vi "Get Data and Log.vi"() -> ()   [LabVIEW 2016]
uses:
  <vilib>/Utility/sysdir.llb/System Directory Type.ctl
  <vilib>/Rock Robotics/Network Tables/NT Read Numeric Array.vi
  <vilib>/Utility/file.llb/Write Delimited Spreadsheet (DBL).vi
panel:
  in  "Mode":T1(ring)=enum."Auto Disabled"
  out "appended path":path
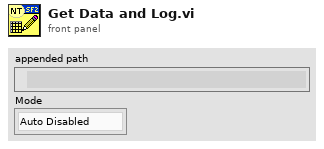
[diagram p1: front panel]
types:
  T1 = enum8{"Tele-Op Disabled", "Tele-Op Enabled", "Auto Disabled", "Auto Enabled", "Test Disabled", "Test Enabled", "Disconnected", "No Code", "E-Stop"}
  T2 = enum16{"open", "replace", "create", "open or create", "replace or create", "replace or create with confirmation"}
  T3 = typedef "System Directory Type.ctl" = i32
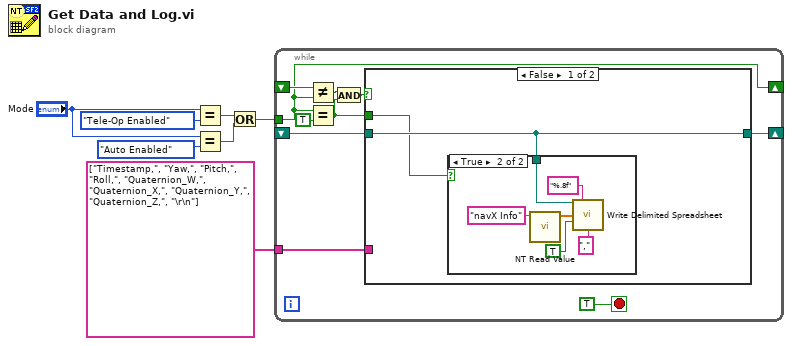
[diagram p0: block diagram]
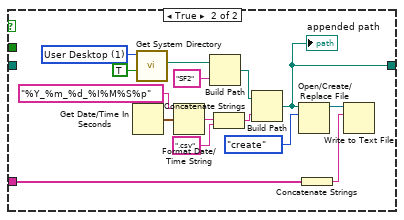
[diagram p3: hidden frame]
diagram:
  n1 = Equal?(x="Mode", y=T1."Tele-Op Enabled") -> (x = y?=w4:bool)
  n2 = Equal?(x="Mode", y=T1."Auto Enabled") -> (x = y?=w3:bool)
  n3 = Or(x=w4, y=w3) -> (x .or. y?=w2:bool)
  n4 = while {
    shift-right: [w15] -> _
    shift-left: _ -> [w16]
    tunnel: w2 -> [w12]
    shift-right: [w12] -> _
    shift-left: _ -> [w14]
    tunnel: string[] ["Timestamp,", "Yaw,", "Pitch,", "Roll,", "Quaternion_W,", "Quaternion_X,", "Quaternion_Y,", "Quaternion_Z,", "\r\n"] -> [w8]
    stop <- TRUE stop-if-true
    n5 = Not Equal?(x=w14, y=w12) -> (x != y?=w13:bool)
    n6 = Equal?(x=w12, y=TRUE) -> (x = y?=w9:bool)
    n7 = And(x=w13, y=w9) -> (x .and. y?=w10:bool)
    n8 = case shown="False" w10 {
      tunnel: [w19 w26] -> w15
      tunnel: w16 -> [w19 _]
      tunnel: w9 -> [w18 _]
      tunnel: w8 -> [_ w31]
      frame False {
        n9 = case shown="True" w18 {
          tunnel: w19 -> [_ w22]
          frame False {
          }
          frame True {
            n10 = call-poly <vilib>:"NT Read Value.vi"("Name"="navX Info") -> ("Numeric Array"=w21:dbl[])  [unwired: 9 in, 1 out]
            n11 = call-poly <vilib>:"Write Delimited Spreadsheet.vi"("file path (dialog if empty)"=w22, "format (%.3f)"="%.8f", "1D data"=w21, "append to file? (new file:F)"=TRUE, "delimiter (\\t)"="," ("delimiter (\\t)")) -> ()  [unwired: 9 in, 2 out]
          }
        }
      }
      frame True {
        w36 = T3 1 items=["User Home"=0, "User Desktop"=1, "User Documents"=2, "User Application Data"=3, "User Preferences"=4, "User Temporary"=5, "Public Documents"=6, "Public Application Data"=7, "Public Preferences"=8, "Public Cache"=13, "System Core Libraries"=9, "System Installed Libraries"=10, "Application Files"=11, "Boot Volume Root"=12] ("system directory type")
        n12 = Get Date/Time In Seconds() -> (seconds since 1Jan1904=w40:timestamp)
        n13 = call <vilib>:"Get System Directory.vi"("create directory if not found? (F)"=TRUE, "system directory type"=w36) -> ("system directory"=w35:path)  [unwired: 9 in]
        n14 = Format Date/Time String(time format string (%c)="%Y_%m_%d_%I%M%S%p", seconds (now)=w40) -> (date/time string=w30:string)  [unwired: 1 in]
        n15 = Build Path(base path=w35, name or relative path="SF2") -> (appended path=w32:path)
        n16 = Concatenate Strings(w30, ".csv" ("string")) -> (w28:string)
        n17 = Build Path(base path=w32, name or relative path=w28) -> (appended path=w26:path)
        "appended path" <- w26
        n18 = Open/Create/Replace File(file path (use dialog)=w26, operation (0:open)=T2."create") -> (refnum out=w38:refnum<file>)  [unwired: 4 in, 2 out]
        n19 = Concatenate Strings(w31) -> (w27:string)
        n20 = Write to Text File(file (use dialog)=w38, text=w27) -> ()  [unwired: 2 in, 3 out]
      }
    }
  }
